vi "Register Existing String Item.vi"(8 "error in (no error)":errorcluster, 9 "notifier in":refnum<notifier>, 10 "Tag Name":string, 11 "Current Value Table in":refnum<class "Current Value Table.lvclass">) -> (0 "error out":errorcluster, 3 "Current Value Table out":refnum<class "Current Value Table.lvclass">)   [LabVIEW 2024, in "Current Value Table.lvlib" / "Current Value Table.lvclass"]
uses:
  Current Value Table.lvclass
  CVT_String/CVT_String.lvclass
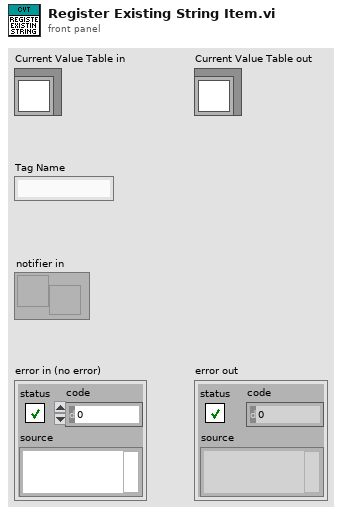
[diagram p1: front panel]
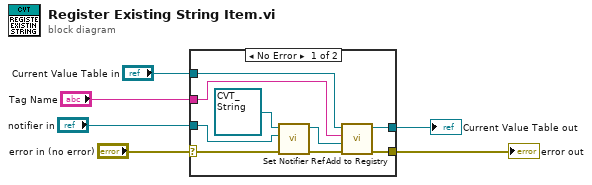
[diagram p0: block diagram]
diagram:
  n1 = case shown="No Error" "error in (no error)" {
    selector: "error in (no error)" -> [w13 w17]
    tunnel: [w7 w17] -> w5
    tunnel: [w8 w16] -> w3
    tunnel: "Current Value Table in" -> [w9 w16]
    tunnel: "notifier in" -> [w14 _]
    tunnel: "Tag Name" -> [w12 _]
    frame No Error {
      n2 = call-dynamic "Set Notifier Ref.vi"("error in (no error)"=w13, "notifier in"=w14, "CVT_String in"=refnum<class "CVT_String.lvclass"> refnum) -> ("error out"=w10:errorcluster, "CVT_String out"=w11:refnum<class "CVT_String.lvclass">)  [unwired: 7 in]
      n3 = call-dynamic "Add to Registry.vi"("error in (no error)"=w10, "iCVT_Item in"=w11, "Tag Name"=w12, "Current Value Table in"=w9) -> ("error out"=w7:errorcluster, "Current Value Table out"=w8:refnum<class "Current Value Table.lvclass">)  [unwired: 5 in, 1 out]
    }
    frame Error {
    }
  }
  "error out" <- w5
  "Current Value Table out" <- w3
